vi "Error Process.vi"(8 "error in (no error)":errorcluster, 11 "View Model":T1) -> (0 "error out":errorcluster)   [LabVIEW 2017]
doc: "Provide all operations for processing all error's types. Centralized Error Handler."
uses:
  View Model/Controls/View Model.ctl
  Configuration/Controls/Config Model.ctl
  Configuration/Controls/Config Data.ctl
  Controls/Error Model.ctl
  Controls/Error Data.ctl
  Controls/Error Type.ctl
  View Model/Controls/Shared Model.ctl
  Elevator Controller/Controls/Elevator Model.ctl
  Elevator Controller/Controls/Elevator Location.ctl
  Elevator Controller/Controls/Elevator CMD Data.ctl
  Elevator Controller/Controls/Elevator Commands.ctl
  Elevator Controller/Controls/Elevator Overhead.ctl
  Elevator Controller/Controls/Elevator States.ctl
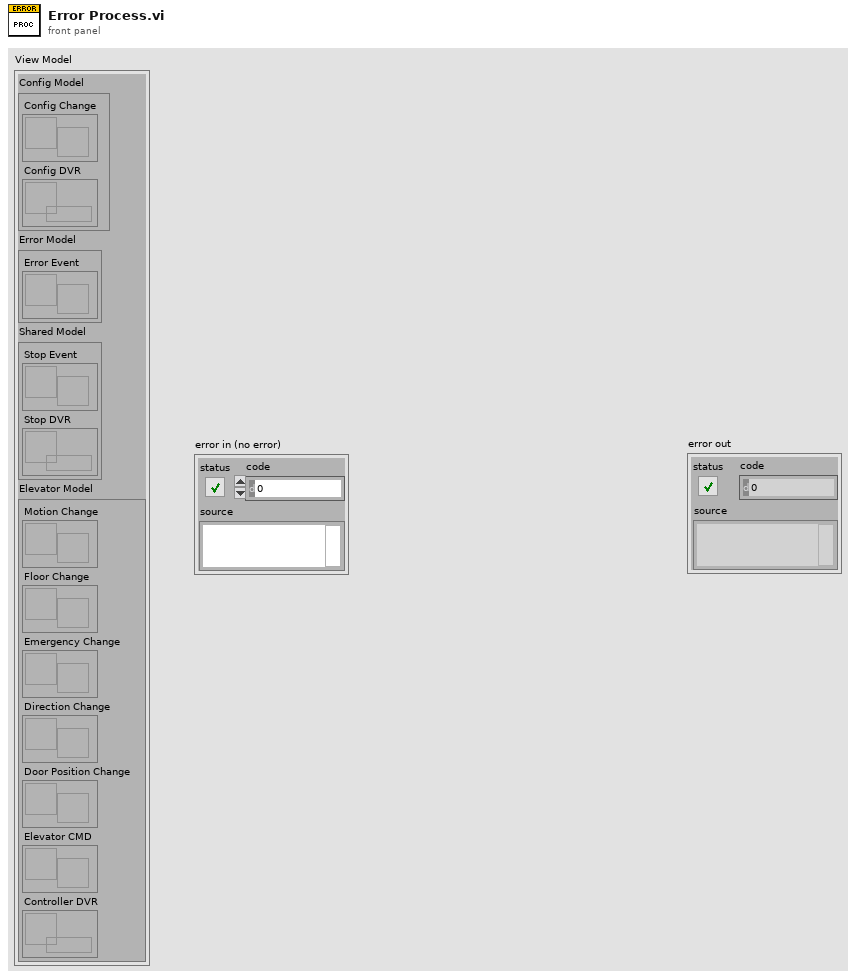
[diagram p1: front panel]
types:
  T1 = typedef "View Model.ctl" = cluster{"Config Model":T2, "Error Model":T3, "Shared Model":T4, "Elevator Model":T5}
  T2 = typedef "Config Model.ctl" = cluster{"Config Change":refnum<user-event>, "Config DVR":refnum<data-value>}
  T3 = typedef "Error Model.ctl" = cluster{"Error Event":refnum<user-event>}
  T4 = typedef "Shared Model.ctl" = cluster{"Stop Event":refnum<user-event>, "Stop DVR":refnum<data-value>}
  T5 = typedef "Elevator Model.ctl" = cluster{"Motion Change":refnum<user-event>, "Floor Change":refnum<user-event>, "Emergency Change":refnum<user-event>, "Direction Change":refnum<user-event>, "Door Position Change":refnum<user-event>, "Elevator CMD":refnum<user-event>, "Controller DVR":refnum<data-value>}
  T6 = typedef "Error Data.ctl" = cluster{"Error Type":T7, "Variant":variant}
  T7 = typedef "Error Type.ctl" = enum16{"Console Error", "Sensor Interface IO Error", "Process Step Error"}
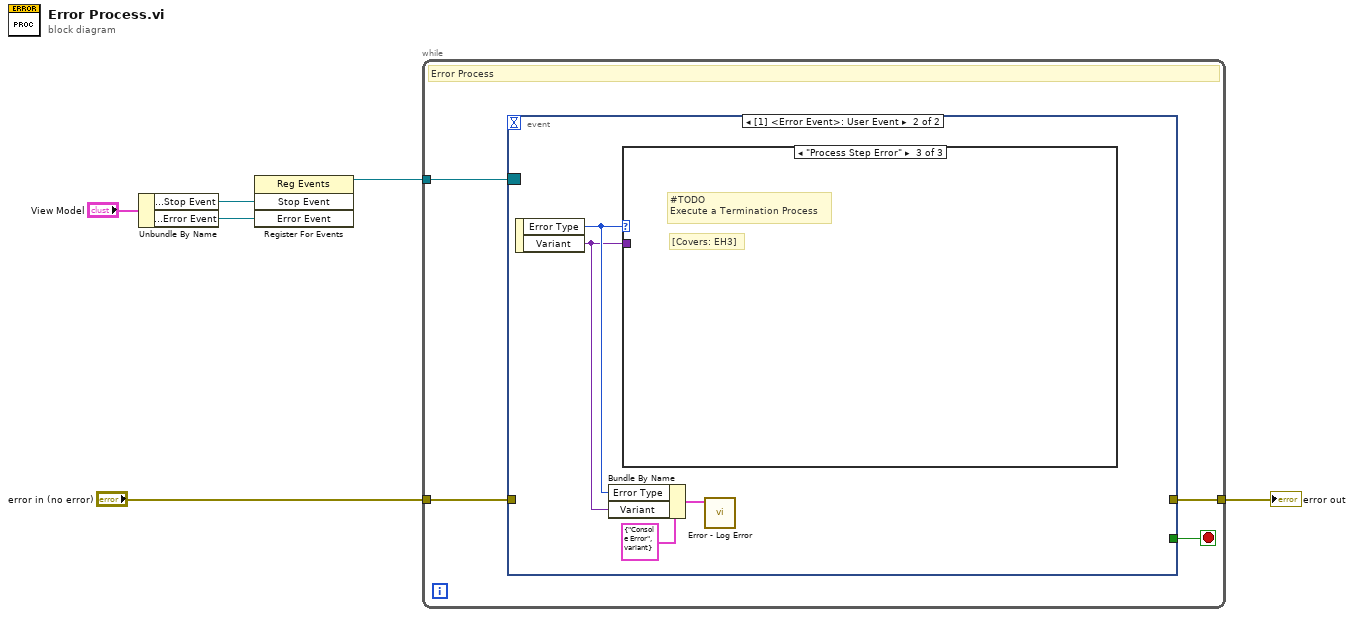
[diagram p0: block diagram]
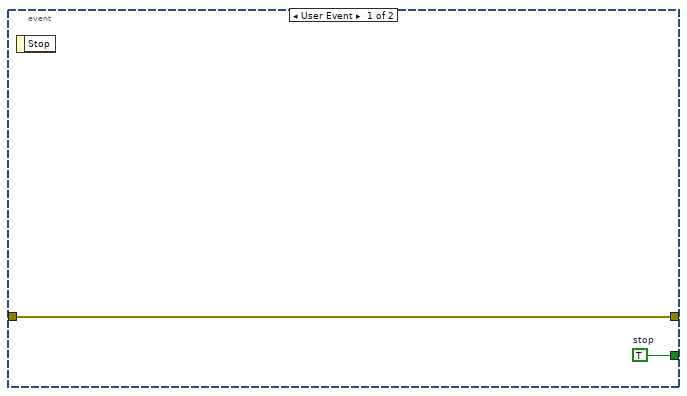
[diagram p2: hidden frame]
diagram:
  n1 = Unbundle By Name("View Model") -> ("Shared Model.Stop Event"=w6:refnum<user-event>, "Error Model.Error Event"=w1:refnum<user-event>)
  n2 = register-events(w6, w1) -> (reference out=w5:refnum<event-registration>)  [unwired: 2 in, 1 out]
  n3 = while {
    tunnel: w5 -> [w10]
    tunnel: "error in (no error)" -> [w8]
    tunnel: [w7] -> w3
    stop <- w9 stop-if-true
    # "Error Process"
    n4 = event shown="[1] <Error Event>: User Event" {
      selector: w10 -> [_ _]
      dyn-events: _ -> [_ _]
      timeout: _ -> [_ _]
      tunnel: [w12 _] -> w9
      tunnel: w8 -> [w11 _]
      tunnel: [w11 _] -> w7
      event User Event {
        w12 = TRUE  # stop
        n5 = event-data() -> ()  [unwired: 1 in, 1 out]
      }
      event User Event {
        n6 = event-data() -> ("Error Type"=w15:T7, "Variant"=w14:variant)  [unwired: 1 in]
        n7 = Bundle By Name(cluster=T6 {"Error Type"=enum."Console Error", "Variant"=variant} ("Error Data"), "Error Type"=w15, "Variant"=w14) -> (w13:T6)
        n8 = case shown="\"Process Step Error\"" w15 {
          tunnel: w14 -> [_ _ _]
          frame "Console Error", Default {
            # "[Covers: EH1B2]"
            # "[Covers: EH1B1]"
            # "[Covers: EH1B]"
            # "[Covers: EH1A]"
            # "#TODO\nIf error source = Display Console View, notify user and clear error\n\nIf error source = User Console View, Allow user to choose to clear\nor continue w/error.\n- If error cleared, continue last operation.\n- If continue, process error as a \"Process Step Error\""
            # "[Covers: EH1]"
            # "#TODO\nNotify User about Error adn continue operations without interruption"
          }
          frame "Sensor Interface IO Error" {
            # "[Covers: EH2]"
            # "#TODO\nExecute a Termination Process"
          }
          frame "Process Step Error" {
            # "[Covers: EH3]"
            # "#TODO\nExecute a Termination Process"
          }
        }
        n9 = call "Error - Log Error.vi"("Error Data"=w13) -> ()  [unwired: 10 in, 1 out]
      }
    }
  }
  "error out" <- w3
